vi "Thermocouple.vi"(11 "Queue ref":T1) -> ()   [LabVIEW 2022 SP3]
uses:
  Controls/All Queue.ctl
  Controls/DAQ case.ctl
  Controls/All Loop Status.ctl
  <vilib>/DAQmx/read.llb/DAQmx Read (Analog 1D Wfm NChan NSamp).vi
  Create Task/TC Create Task.vi
  <vilib>/DAQmx/configure/timing.llb/DAQmx Timing (Sample Clock).vi
  Sub VI's/Global 1.vi
  <vilib>/DAQmx/miscellaneous.llb/DAQmx Fill In Error Info.vi
panel:
  # "TC channel list"
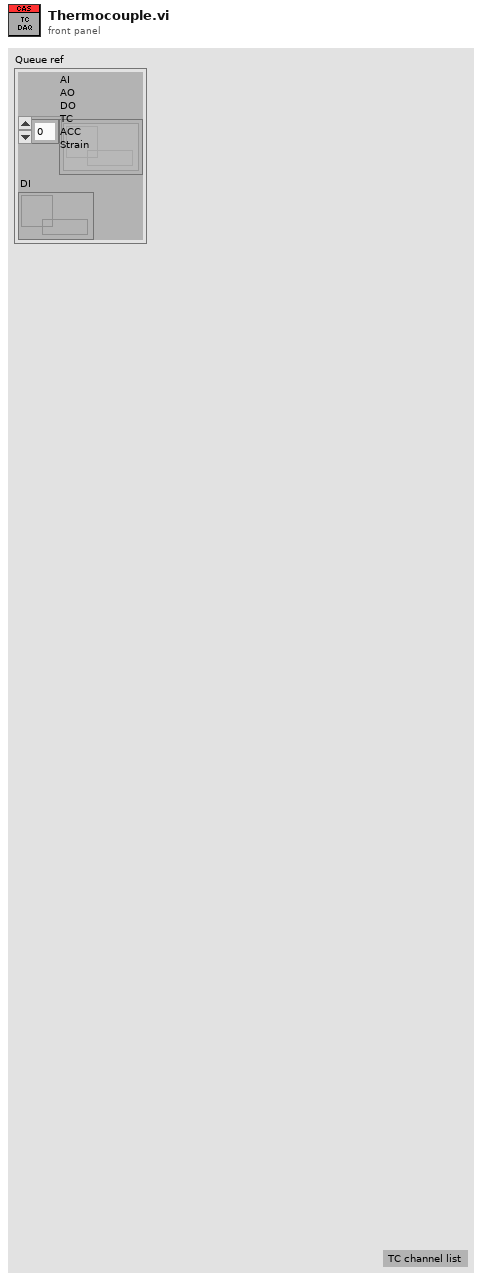
[diagram p1: front panel]
types:
  T1 = typedef "All Queue.ctl" = cluster{"AI\nAO\nDO\nTC\nACC\nStrain":refnum<queue>[], "DI":refnum<queue>}
  T2 = cluster{"in progress?":bool, "Queue ref":T1, "Start DAQ":refnum<notifier>, "task out":refnum<k21>, "TC Ref":refnum<queue>, "SPC":i32}
  T3 = typedef "DAQ case.ctl" = enum16{"Initailise", "Create Task", "Polevent", "Acquire", "Stop DAQ", "Error", "Exit"}
  T4 = typedef "All Loop Status.ctl" = enum16{"AI", "AO", "DI", "DO", "TC", "Strain", "ACC", "RT", "Log"}
  T5 = enum16{"Init", "Read 'All'", "Read 'n'", "Read '1'", "Write '1'", "Write 'n'", "Write 'All'"}
  T6 = typedef "All Notifer.ctl" = cluster{"UI Data":refnum<notifier>, "Start DAQ":refnum<notifier>, "Start Log":refnum<notifier>}
  T7 = cluster{"Analog input":bool, "Analog Output":bool, "Digital input":bool, "Digital output":bool, "Thermocouple":bool, "Strain Gauge":bool, "Accelerometer":bool}
  T8 = typedef "Config.ctl" = cluster{"AO config":cluster{"Channel_Name":string, "Channel_Number":string, "Default_Value":dbl, "Units":string}[], "AI config":cluster{"Channel_Name":string, "Channel_Number":string, "Pre_Scale_min":dbl, "Pre_Scale_max":dbl, "Sensor_min":dbl, "Sensor_max":dbl, "Units":string}[], "DI config":cluster{"Channel_Name":string, "Channel_Number":string, "Default_Value":bool, "DI invert?":bool}[], "DO config":cluster{"Channel_Name":string, "Channel_Number":string, "Default_Value":bool, "DO invert?":bool}[], "TC config":cluster{"Channel_Name":string, "Channel_Number":string, "Pre_Scale_min":dbl, "Pre_Scale_max":dbl, "units":i32, " type":i32}[], "ACC config":cluster{"Channel_Name":string, "Channel_Number":string, "Pre_Scale_min":dbl, "Pre_Scale_max":dbl, "Terminal configuration":i32, "Sensitivity":dbl, "Sensitivity units":i32}[], "SG config":cluster{"Channel_Name":string, "Channel_Number":string, "Pre_Scale_min":dbl, "Pre_Scale_max":dbl}[], "Strain Gauge Settings":cluster{"poisson ratio":dbl, "nominal gage resistance":dbl, "gage factor":dbl}, "bridge information":cluster{"strain configuration":i32, "lead wire resistance":dbl, "initial bridge voltage":dbl, "voltage excitation source":i32, "voltage excitation value":dbl}, "Sample Rate":cluster{"AI Sample Rate":dbl, "AO Sample Rate":dbl, "DI Sample Rate":dbl, "TC Sample Rate":dbl, "DO Sample Rate":dbl, "SG Sample Rate":dbl, "ACC Sample Rate":dbl}}
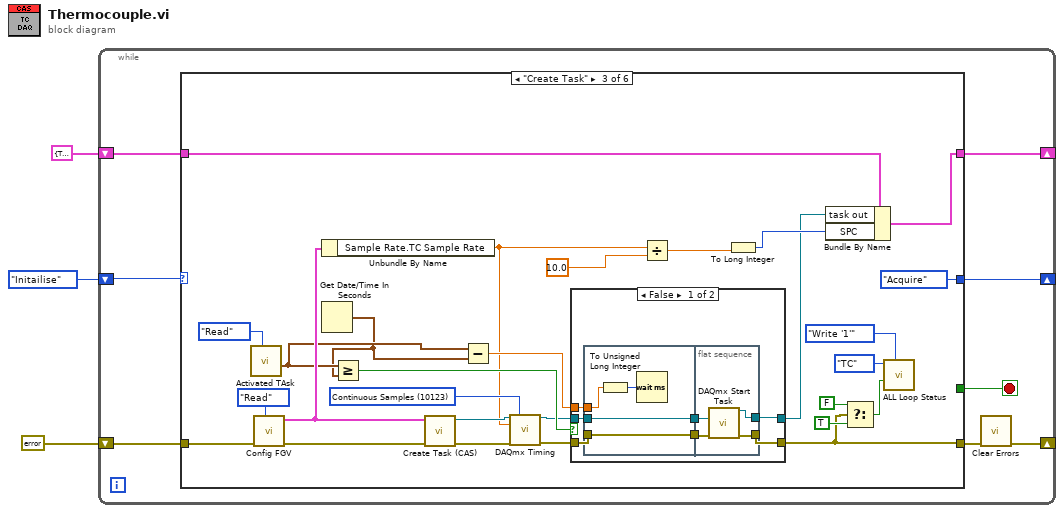
[diagram p0: block diagram]
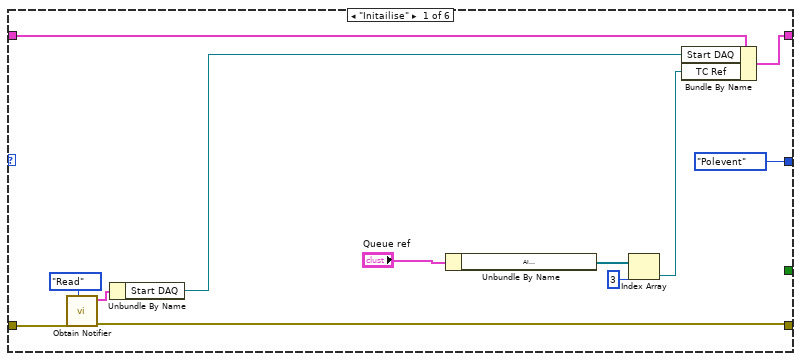
[diagram p2: hidden frame]
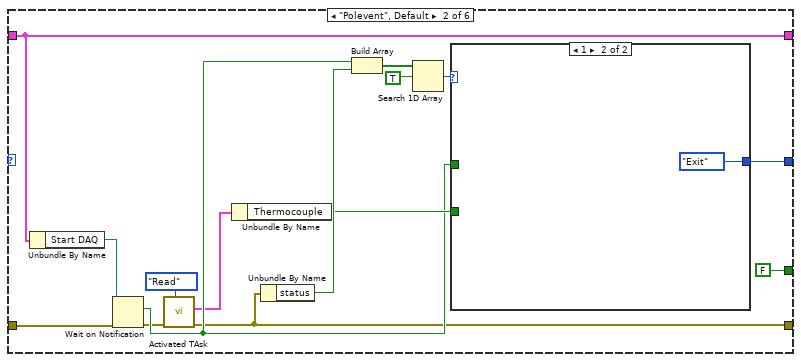
[diagram p3: hidden frame]
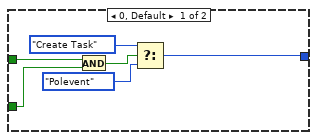
[diagram p4: hidden frame]
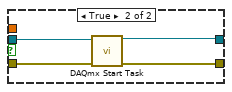
[diagram p5: hidden frame]
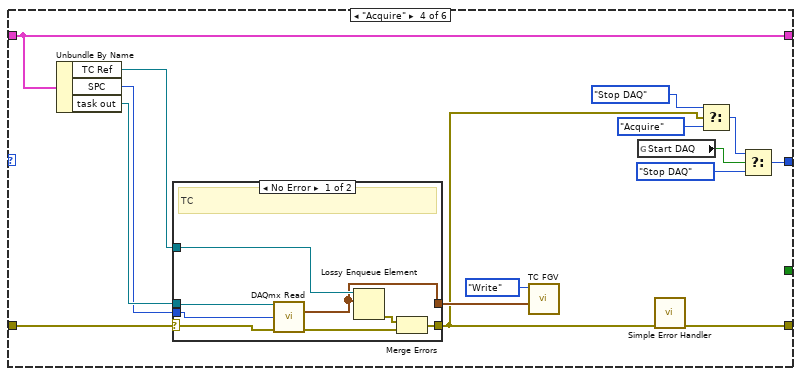
[diagram p6: hidden frame]
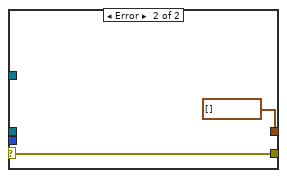
[diagram p7: hidden frame]
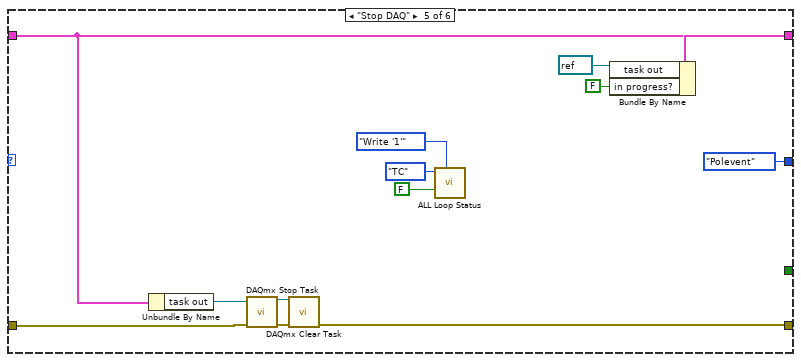
[diagram p8: hidden frame]
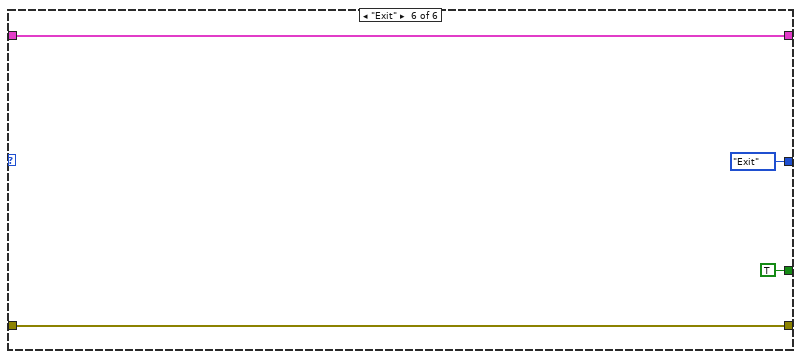
[diagram p9: hidden frame]
diagram:
  n1 = while {
    shift-right: [w4] -> _
    shift-left: errorcluster {"status"=FALSE, "code"=0, "source"=""} ("error out") -> [w10]
    shift-right: [w8] -> _
    shift-left: T2 {"in progress?"=TRUE, "Queue ref"={"AI\nAO\nDO\nTC\nACC\nStrain"=[], "DI"=refnum}, "Start DAQ"=refnum, "task out"="", "TC Ref"=refnum, "SPC"=0} -> [w9]
    shift-right: [w7] -> _
    shift-left: DAQ_case."Initailise" -> [w6]
    stop <- w11 stop-if-true
    n2 = case shown="\"Create Task\"" w6 {
      tunnel: [_ FALSE _ _ _ TRUE] -> w11
      tunnel: w10 -> [w22 w27 w70 w100 w122 w134]
      tunnel: [w21 w25 w52 w95 w123 w134] -> w5
      tunnel: w9 -> [w19 w36 w72 w101 w127 w133]
      tunnel: [w17 w36 w71 w101 w128 w133] -> w8
      tunnel: [DAQ_case."Polevent" w37 DAQ_case."Acquire" w102 DAQ_case."Polevent" DAQ_case."Exit"] -> w7
      frame "Initailise" {
        n3 = call "Obtain Notifier.vi"("Case"=enum16{"Obtain", "Read"}."Read", "error in (no error)"=w22) -> ("error out"=w21:errorcluster, "notifiers out"=w20:T6)  [unwired: 8 in]
        n4 = Unbundle By Name(w20) -> ("Start DAQ"=w18:refnum<notifier>)
        n5 = Unbundle By Name("Queue ref") -> ("AI\nAO\nDO\nTC\nACC\nStrain"=w14:refnum<queue>[])
        n6 = Index Array(array=w14, index=3) -> (element=w13:refnum<queue>)
        n7 = Bundle By Name(cluster=w19, "Start DAQ"=w18, "TC Ref"=w13) -> (w17:T2)
      }
      frame "Polevent", Default {
        n8 = Unbundle By Name(w36) -> ("Start DAQ"=w35:refnum<notifier>)
        n9 = Wait on Notification(notifier=w35, error in (no error)=w27) -> (notification=w28:bool, error out=w26:errorcluster)  [unwired: 2 in, 2 out]
        n10 = call "Activated TAsk.vi"("Enum"=enum16{"Read", "Write"}."Read", "error in (no error)"=w26) -> ("error out"=w25:errorcluster, "Activate Task 2"=w24:T7)  [unwired: 7 in, 1 out]
        n11 = Unbundle By Name(w24) -> ("Thermocouple"=w29:bool)
        n12 = Unbundle By Name(w25) -> ("status"=w34:bool)
        n13 = Build Array(w28, w34) -> (w33:bool[])
        n14 = Search 1D Array(1D array=w33, element=TRUE) -> (index of element=w31:i32)  [unwired: 1 in]
        n15 = case shown="1" w31 {
          tunnel: [w43 DAQ_case."Exit"] -> w37
          tunnel: w29 -> [w40 _]
          tunnel: w28 -> [w39 _]
          frame 0, Default {
            n16 = And(x=w39, y=w40) -> (x .and. y?=w41:bool)
            n17 = Select(t=DAQ_case."Create Task", s=w41, f=DAQ_case."Polevent") -> (s? t:f=w43:T3)
          }
          frame 1 {
          }
        }
      }
      frame "Create Task" {
        w65 = 10123 items=["Finite Samples"=10178, "Continuous Samples"=10123, "Hardware Timed Single Point"=12522] ("sample mode")
        n18 = call "Activated TAsk.vi"("Enum"=enum16{"Read", "Write"}."Read") -> ("Start Time"=w50:timestamp)  [unwired: 8 in, 2 out]
        n19 = call "Config FGV.vi"("Enum"=enum16{"Read", "Write"}."Read", "error in (no error)"=w70) -> ("error out"=w67:errorcluster, "Data"=w59:T8)  [unwired: 8 in]
        n20 = Unbundle By Name(w59) -> ("Sample Rate.TC Sample Rate"=w48:dbl)
        n21 = Get Date/Time In Seconds() -> (seconds since 1Jan1904=w49:timestamp)
        n22 = Greater Or Equal?(x=w50, y=w49) -> (x >= y?=w54:bool)
        n23 = call-poly "Create Task (CAS).vi"("error in"=w67, "config"=w59) -> ("error out"=w66:errorcluster, "task out"=w58:refnum<k21>)  [unwired: 7 in, 1 out]
        n24 = Subtract(x=w50, y=w49) -> (x-y=w56:dbl)
        n25 = call-poly <vilib>:"DAQmx Timing.vi"("task/channels in"=w58, "sample mode"=w65, "rate"=w48, "error in"=w66) -> ("task out"=w53:refnum<k21>, "error out"=w55:errorcluster)  [unwired: 10 in]
        n26 = case shown="False" w54 {
          tunnel: w55 -> [w80 w92]
          tunnel: [w79 w91] -> w52
          tunnel: w53 -> [w78 w89]
          tunnel: [w77 w90] -> w51
          tunnel: w56 -> [w74 _]
          frame False {
            n27 = flat-sequence {
              tunnel: w78 -> [w83]
              tunnel: w80 -> [w84]
              tunnel: [w84] -> w76
              tunnel: [w83] -> w75
              tunnel: w74 -> [w81]
              tunnel: [w87] -> w79
              tunnel: [w85] -> w77
              tunnel: w76 -> [w88]
              tunnel: w75 -> [w86]
              frame #0 {
                n28 = To Unsigned Long Integer(number=w81) -> (unsigned 32bit integer=w82:u32)
                n29 = Wait (ms)(milliseconds to wait=w82) -> ()  [unwired: 1 out]
              }
              frame #1 {
                n30 = call <vilib>:"DAQmx Start Task.vi"("task/channels in"=w86, "error in"=w88) -> ("task out"=w85:refnum<k21>, "error out"=w87:errorcluster)  [unwired: 12 in]
              }
            }
          }
          frame True {
            n31 = call <vilib>:"DAQmx Start Task.vi"("task/channels in"=w89, "error in"=w92) -> ("task out"=w90:refnum<k21>, "error out"=w91:errorcluster)  [unwired: 12 in]
          }
        }
        n32 = Divide(x=w48, y=10.0) -> (x/y=w47:dbl)
        n33 = To Long Integer(number=w47) -> (32bit integer=w57:i32)
        n34 = Bundle By Name(cluster=w72, "task out"=w51, "SPC"=w57) -> (w71:T2)
        n35 = Select(t=FALSE, s=w52, f=TRUE) -> (s? t:f=w62:bool)
        n36 = call "ALL Loop Status.vi"("Option"=T5."Write '1'", "Status"=w62, "Loop"=All_Loop_Status."TC") -> ()  [unwired: 6 in, 3 out]
      }
      frame "Acquire" {
        n37 = Unbundle By Name(w101) -> ("TC Ref"=w94:refnum<queue>, "SPC"=w93:i32, "task out"=w99:refnum<k21>)
        n38 = case shown="No Error" w100 {
          selector: w100 -> [w111 w117]
          tunnel: w99 -> [w110 _]
          tunnel: [w113 w117] -> w96
          tunnel: w94 -> [w112 _]
          tunnel: [w109 waveform(dbl)[] [] ("data")] -> w97
          tunnel: w93 -> [w108 _]
          frame No Error {
            # "TC"
            n39 = call-poly <vilib>:"DAQmx Read.vi"("task/channels in"=w110, "number of samples per channel"=w108, "error in"=w111) -> ("data"=w109:waveform(dbl)[], "error out"=w114:errorcluster)  [unwired: 10 in, 1 out]
            n40 = Lossy Enqueue Element(queue=w112, element=w109) -> (error out=w115:errorcluster)  [unwired: 1 in, 3 out]
            n41 = Merge Errors(w115, w114) -> (w113:errorcluster)
          }
          frame Error {
          }
        }
        n42 = call "TC FGV.vi"("AI data"=w97, "Enum"=enum16{"Read", "Write"}."Write") -> ()  [unwired: 9 in, 1 out]
        n43 = global read "Global 1.vi" "Start DAQ"() -> (w105:bool)
        n44 = call <vilib>:"Simple Error Handler.vi"("error in (no error)"=w96) -> ("error out"=w95:errorcluster)  [unwired: 4 in, 4 out]
        n45 = Select(t=DAQ_case."Stop DAQ", s=w96, f=DAQ_case."Acquire") -> (s? t:f=w104:T3)
        n46 = Select(t=w104, s=w105, f=DAQ_case."Stop DAQ") -> (s? t:f=w102:T3)
      }
      frame "Stop DAQ" {
        n47 = Unbundle By Name(w127) -> ("task out"=w121:refnum<k21>)
        n48 = call <vilib>:"DAQmx Stop Task.vi"("task/channels in"=w121, "error in"=w122) -> ("task out"=w120:refnum<k21>, "error out"=w124:errorcluster)  [unwired: 12 in]
        n49 = call <vilib>:"DAQmx Clear Task.vi"("task in"=w120, "error in"=w124) -> ("error out"=w123:errorcluster)  [unwired: 13 in]
        n50 = call "ALL Loop Status.vi"("Option"=T5."Write '1'", "Status"=FALSE, "Loop"=All_Loop_Status."TC") -> ()  [unwired: 6 in, 3 out]
        n51 = Bundle By Name(cluster=w127, "task out"=refnum<k21> refnum, "in progress?"=FALSE) -> (w128:T2)
      }
      frame "Exit" {
      }
    }
    n52 = call <vilib>:"Clear Errors.vi"("error in (no error)"=w5) -> ("error out"=w4:errorcluster)  [unwired: 5 in, 1 out]
  }
